vi "Configure Hardware.vi"(8 "error in (no error)":errorcluster, 11 "Hardware Resources in":T1={"DAQmx Channel"="", "Sample Rate"=0.0, "DAQmx Task"="", "ResetInterp"=FALSE, "GainConstants"=[2.0, 10.0, 1.0, 0.1, 0.01, 0.001], "FilterCoefficients"=[], "ChannelNames"=[], "ActiveChannels"=[], "Display Rate"=1000, "ResponseExtension"=TRUE}) -> (0 "error out":errorcluster, 3 "Hardware Resources out":T1={"DAQmx Channel"="", "Sample Rate"=0.0, "DAQmx Task"="", "ResetInterp"=FALSE, "GainConstants"=[2.0, 10.0, 1.0, 0.1, 0.01, 0.001], "FilterCoefficients"=[], "ChannelNames"=[], "ActiveChannels"=[], "Display Rate"=1000, "ResponseExtension"=TRUE})   [LabVIEW 2017, in "Acquisition.lvlib"]
doc: "Configure the hardware."
uses:
  Acquisition.lvlib
  Hardware Configuration.ctl
  <vilib>/DAQmx/create/channels.llb/DAQmx Create Channel (AI-Voltage-Basic).vi
  <vilib>/DAQmx/configure/timing.llb/DAQmx Timing (Sample Clock).vi
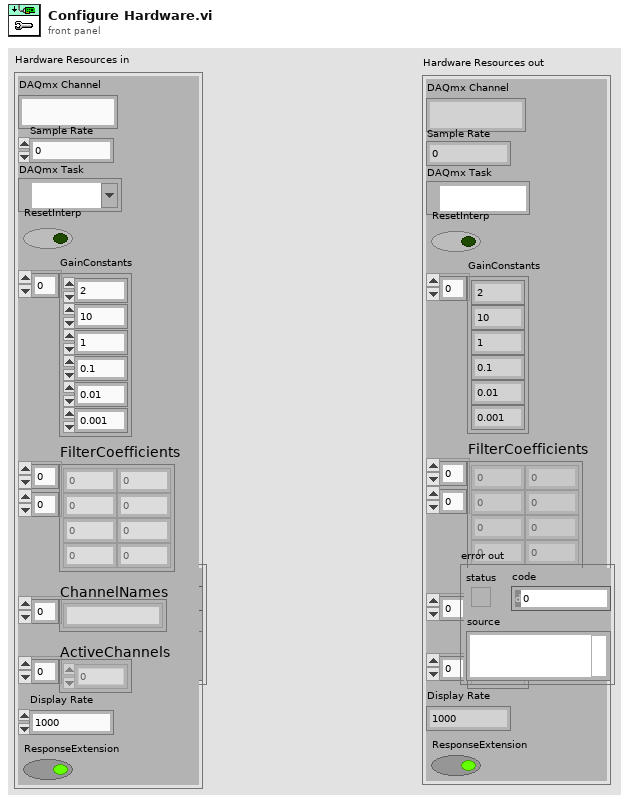
[diagram p1: front panel]
types:
  T1 = typedef "Acquisition.lvlib/Hardware Configuration.ctl" = cluster{"DAQmx Channel":string, "Sample Rate":dbl, "DAQmx Task":refnum<k21>, "ResetInterp":bool, "GainConstants":dbl[], "FilterCoefficients":dbl[][], "ChannelNames":string[], "ActiveChannels":i32[], "Display Rate":i32, "ResponseExtension":bool}
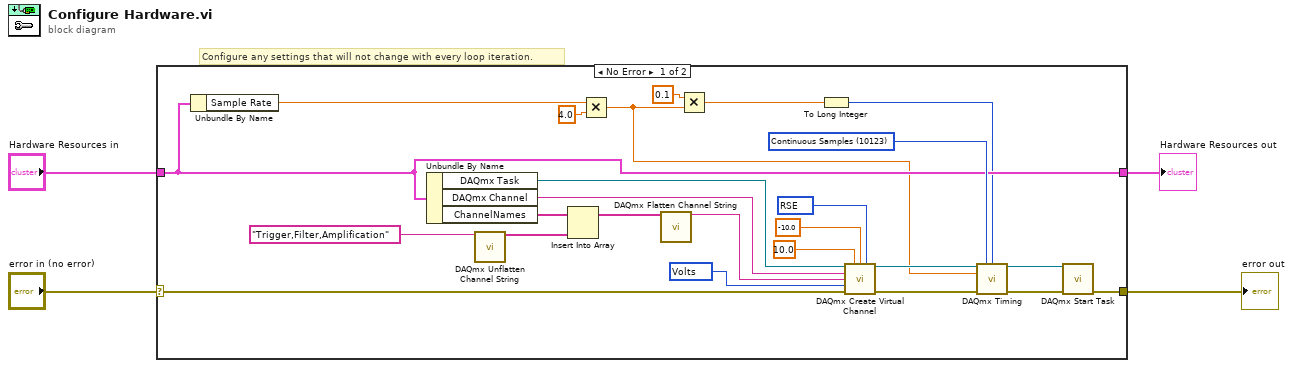
[diagram p0: block diagram]
diagram:
  # "Configure any settings that will not change with every loop iteration."
  n1 = case shown="No Error" "error in (no error)" {
    selector: "error in (no error)" -> [w26 w30]
    tunnel: [w24 w30] -> w3
    tunnel: "Hardware Resources in" -> [w16 w31]
    tunnel: [w16 w31] -> w1
    frame No Error {
      w21 = 10083 items=["Default"=-1, "RSE"=10083, "NRSE"=10078, "Differential"=10106, "Pseudodifferential"=12529] ("input terminal configuration")
      w23 = 10348 items=["Volts"=10348, "From Custom Scale"=10065] ("units")
      w25 = 10123 items=["Finite Samples"=10178, "Continuous Samples"=10123, "Hardware Timed Single Point"=12522] ("sample mode")
      n2 = Unbundle By Name(w16) -> ("Sample Rate"=w15:dbl)
      n3 = Unbundle By Name(w16) -> ("DAQmx Task"=w29:refnum<k21>, "DAQmx Channel"=w28:string, "ChannelNames"=w5:string[])
      n4 = call <vilib>:"DAQmx Unflatten Channel String.vi"("names in"="Trigger,Filter,Amplification" ("name to assign")) -> ("names out"=w7:string[])  [unwired: 13 in, 1 out]
      n5 = Insert Into Array(array=w5, new element=w7) -> (w6:string[])  [unwired: 1 in]
      n6 = Multiply(x=w15, y=4.0) -> (x*y=w13:dbl)
      n7 = call <vilib>:"DAQmx Flatten Channel String.vi"("names in"=w6) -> ("names out"=w8:string)  [unwired: 13 in, 1 out]
      n8 = Multiply(x=0.1 ("y"), y=w13) -> (x*y=w11:dbl)
      n9 = To Long Integer(number=w11) -> (32bit integer=w10:i32)
      n10 = call-poly <vilib>:"DAQmx Create Virtual Channel.vi"("task in"=w29, "maximum value"=10.0, "minimum value"=-10.0, "input terminal configuration"=w21, "physical channels"=w28, "name to assign"=w8, "units"=w23, "error in"=w26) -> ("task out"=w22:refnum<k21>, "error out"=w27:errorcluster)  [unwired: 6 in]
      n11 = call-poly <vilib>:"DAQmx Timing.vi"("task/channels in"=w22, "sample mode"=w25, "samples per channel"=w10, "rate"=w13, "error in"=w27) -> ("task out"=w20:refnum<k21>, "error out"=w19:errorcluster)  [unwired: 9 in]
      n12 = call <vilib>:"DAQmx Start Task.vi"("task/channels in"=w20, "error in"=w19) -> ("error out"=w24:errorcluster)  [unwired: 12 in, 1 out]
    }
    frame Error {
    }
  }
  "Hardware Resources out" <- w1
  "error out" <- w3
